vi "Main.vi"() -> ()   [LabVIEW 2020]
uses:
  <vilib>/vision/NI_Vision_Development_Module.lvlib
panel:
  out "FoundGreen":bool
  out "FoundYellow":bool
  out "FoundRed":bool
  in  "停止":bool
  out "Image":T1(plugin-control)
  out "Color Spectrum":dbl[](array[numeric]) format="%.2f"
  in  "Rectangle":T2={"Left"=292, "Top"=176, "Right"=452, "Bottom"=307, "Rotation"=0.0} {"Rotation" min=-90.0 max=90.0 step=1.0 format="%.2f"; "Left" scale=0.0..1024.0; "Right" scale=0.0..1024.0}
  in  "File Path":path
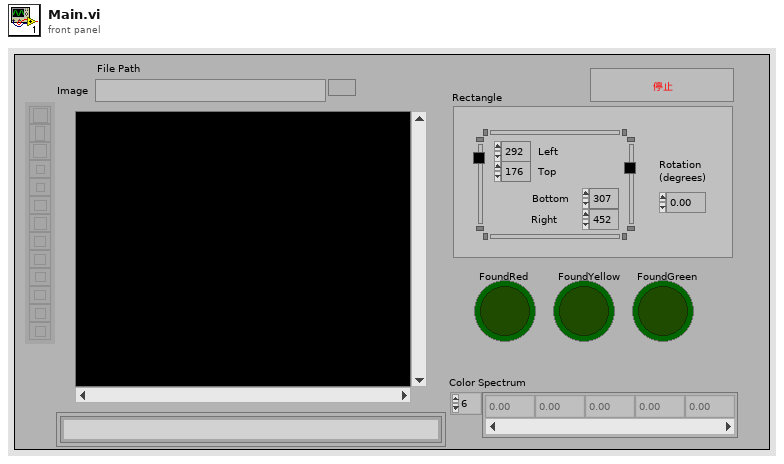
[diagram p1: front panel]
types:
  T1 = typedef "IMAQ Image.ctl" = refnum<image>
  T2 = typedef "IMAQ Rectangle" = cluster{"Left":i32, "Top":i32, "Right":i32, "Bottom":i32, "Rotation":dbl}
  T3 = typedef "ROI Descriptor" = cluster{"Global Rectangle":i32[], "Contours":cluster{"ID":enum32{"External", "Internal"}, "Type":u32, "Coordinates":i32[]}[]}
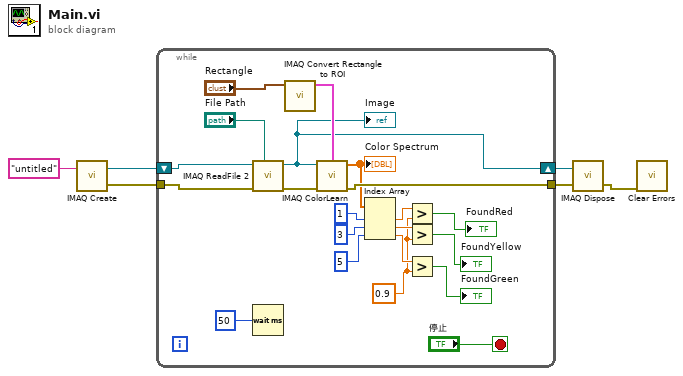
[diagram p0: block diagram]
diagram:
  n1 = call "IMAQ Create"("Image Name"="untitled") -> ("New Image"=w4:T1, "error out"=w5:errorcluster)  [unwired: 4 in]
  n2 = while {
    shift-right: [w21] -> w3
    shift-left: w4 -> [w26]
    tunnel: w5 -> [w25]
    tunnel: [w19] -> w2
    stop <- "停止" stop-if-true
    w9 = 0.9
    n3 = call "IMAQ ReadFile 2"("File Path"="File Path", "error in (no error)"=w25, "Image"=w26) -> ("error out"=w22:errorcluster, "Image Out"=w21:T1)  [unwired: 4 in, 3 out]
    "Image" <- w21
    n4 = Wait (ms)(milliseconds to wait=u32 50 ("等待时间（毫秒）")) -> ()  [unwired: 1 out]
    n5 = call "IMAQ Convert Rectangle to ROI"("Rectangle"="Rectangle") -> ("ROI Descriptor"=w23:T3)  [unwired: 8 in, 1 out]
    n6 = call "IMAQ ColorLearn"("ROI Descriptor"=w23, "Image"=w21, "error in (no error)"=w22) -> ("Color Spectrum"=w17:dbl[], "error out"=w19:errorcluster)  [unwired: 5 in]
    "Color Spectrum" <- w17
    n7 = Index Array(array=w17, index #1=1 ("索引"), index #2=3 ("索引"), index #3=5 ("索引")) -> (element #1=w12:dbl, element #2=w11:dbl, element #3=w10:dbl)
    n8 = Greater?(x=w12, y=w9) -> (0:→"FoundRed":bool)
    n9 = Greater?(x=w11, y=w9) -> (0:→"FoundYellow":bool)
    n10 = Greater?(x=w10, y=w9) -> (0:→"FoundGreen":bool)
  }
  n11 = call "IMAQ Dispose"("Image"=w3, "error in (no error)"=w2) -> ("error out"=w1:errorcluster)  [unwired: 4 in]
  n12 = call <vilib>:"Clear Errors.vi"("error in (no error)"=w1) -> ()  [unwired: 5 in, 2 out]
